vi "API - Transient - Capture Single Transient.vi"(8 "error in":errorcluster, 9 "Data Size":T1, 10 "Maximum Waveform Length":i32=10000, 11 "configuration file path":path) -> (0 "error out":errorcluster)   [LabVIEW 2017, in "DTACQ - Network Enabled Device Driver.lvlib"]
doc: "Captures a single wavelength of data, using the transient capture mode"
uses:
  DTACQ - Network Enabled Device Driver.lvlib
  Communications/Typedefs/Data Size--Enum.ctl
  Close Transient Mode.vi
  Read Transient Data and Write to Shared Variable.vi
  Arm and Fire Transient.vi
  Initialise Transient Mode.vi
  Communications/Communications Library.lvlib
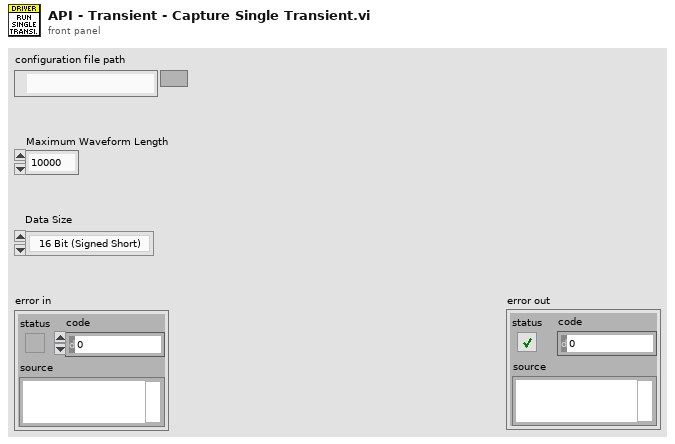
[diagram p1: front panel]
types:
  T1 = typedef "Communications Library.lvlib/Data Size--Enum.ctl" = enum16{"16 Bit (Signed Short)", "32 Bit (Signed Long)"}
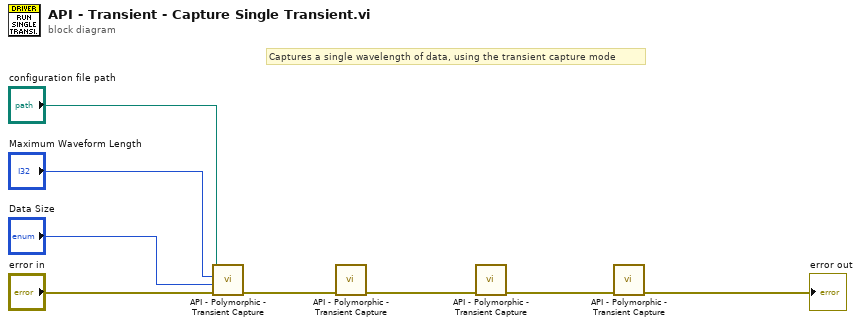
[diagram p0: block diagram]
diagram:
  # "Captures a single wavelength of data, using the transient capture mode"
  n1 = call-poly "API - Polymorphic - Transient Capture.vi"("error in"="error in", "Data Size"="Data Size", "Maximum Waveform Length"="Maximum Waveform Length", "configuration file path"="configuration file path") -> ("error out"=w6:errorcluster)  [unwired: 7 in]
  n2 = call-poly "API - Polymorphic - Transient Capture.vi"("error in"=w6) -> ("error out"=w7:errorcluster)  [unwired: 10 in]
  n3 = call-poly "API - Polymorphic - Transient Capture.vi"("error in"=w7) -> ("error out"=w8:errorcluster)  [unwired: 10 in]
  n4 = call-poly "API - Polymorphic - Transient Capture.vi"("error in"=w8) -> ("error out"=→"error out":errorcluster)  [unwired: 10 in]
